vi "NI-845x Find Devices.vi"(8 "error in (no error)":errorcluster) -> (0 "error out":errorcluster, 2 "devices found string":string, 3 "Devices found array":string[](array[string]))   [LabVIEW 2014, in "DDS.lvclass"]
uses:
  DDS.lvclass
  ni845x.dll
panel:
  out "return type":i32
  out "errors (local display only)":errorcluster
  out "# Devices":u32
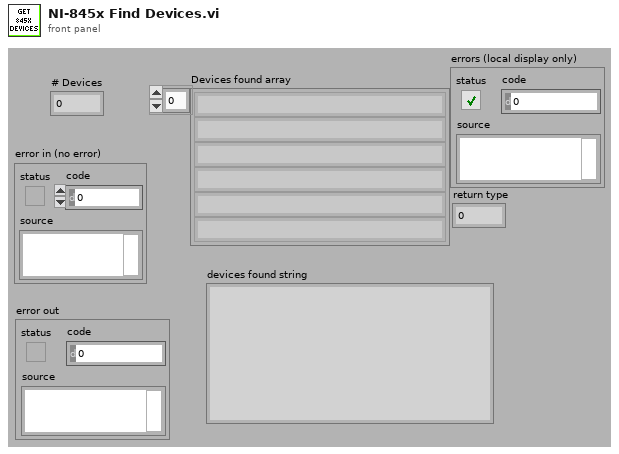
[diagram p1: front panel]
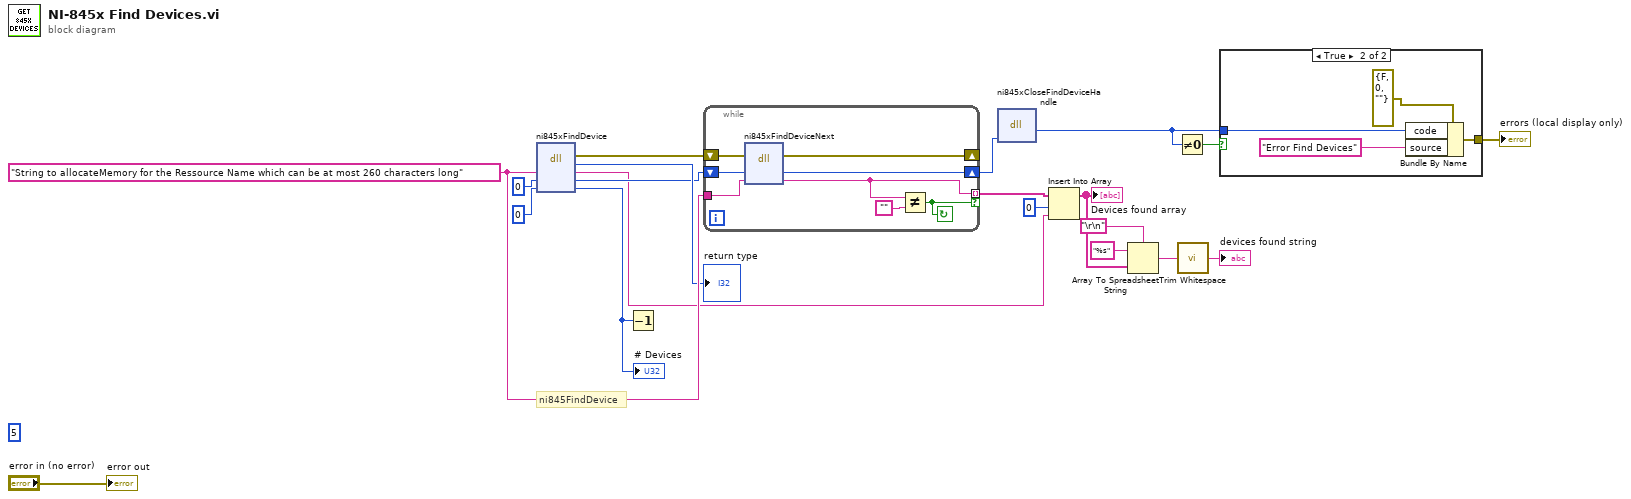
[diagram p0: block diagram]
diagram:
  (unwired) 5
  w16 = "String to allocateMemory for the Ressource Name which can be at most 260 characters long" ("FirstDevice")
  # "ni845FindDevice"
  n1 = dll-call lib="Ni845x.dll" fn="ni845xFindDevice" label="FindDevice"("FirstDevice"=w16, "DeviceHandle"=u32 0, "NumberDevices"=u32 0) -> (error out=w4:errorcluster, "return type"=→"return type":i32, "FirstDevice"=w1:string, "DeviceHandle"=w3:u32, "NumberDevices"=w19:u32)  [unwired: 3 in, 1 out]
  "# Devices" <- w19
  n2 = Decrement(x=w19) -> ()  [unwired: 1 out]
  n3 = while {
    tunnel: [w24] -> w13 mode=indexing if=w23
    tunnel: w16 -> [w26]
    shift-right: [w27] -> w20
    shift-left: w3 -> [w28]
    shift-right: [w21] -> _
    shift-left: w4 -> [w22]
    stop <- w23 continue-if-true
    n4 = dll-call lib="Ni845x.*" fn="ni845xFindDeviceNext"(error in=w22, "FindDeviceHandle"=w28, "pNextDevice"=w26) -> (error out=w21:errorcluster, "FindDeviceHandle"=w27:u32, "pNextDevice"=w24:string)  [unwired: 3 in, 1 out]
    n5 = Not Equal?(x=w24, y="") -> (x != y?=w23:bool)
  }
  n6 = dll-call lib="Ni845x.dll" fn="ni845xCloseFindDeviceHandle"("DeviceHandle"=w20) -> ("return type"=w17:i32)  [unwired: 4 in, 2 out]
  n7 = Insert Into Array(array=w13, index=0, new element=w1) -> (w2:string[])
  "Devices found array" <- w2
  n8 = Array To Spreadsheet String(delimiter (Tab)="\r\n", array=w2, 3:"%s" ("format string")) -> (spreadsheet string=w7:string)
  n9 = Not Equal To 0?(x=w17) -> (x != 0?=w18:bool)
  n10 = call <vilib>:"Trim Whitespace.vi"("string"=w7) -> ("trimmed string"=→"devices found string":string)  [unwired: 1 in]
  n11 = case shown="True" w18 {
    tunnel: w17 -> [_ w32]
    tunnel: [_ w30] -> w11
    frame False {
    }
    frame True {
      n12 = Bundle By Name(cluster=errorcluster {"status"=FALSE, "code"=0, "source"=""} ("error in (no error) 2"), "code"=w32, "source"="Error Find Devices") -> (w30:errorcluster)
    }
  }
  "errors (local display only)" <- w11
  "error out" <- "error in (no error)"
